vi "IO Initial.vi"(8 "error in (no error)":errorcluster, 10 "CardType":u16[](array[ring])=[16, 37] items=["PCI-7230"=6, "PCI-7432"=16, "PCI-7433"=17, "PCI-7434"=18, "PCI-7442"=37]) -> (0 "error out":errorcluster, 2 "IO f":i16[](array[numeric]))   [LabVIEW 2017]
uses:
  <vilib>/Utility/file.llb/Read From Spreadsheet File (string).vi
  Adlink IO/Adlink IO.lvlib
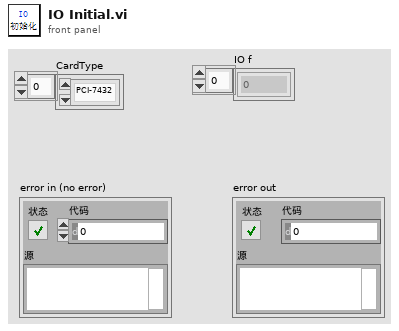
[diagram p1: front panel]
types:
  T1 = cluster{"DI dev":i32[], "DI line":i32[], "Port":i32[], "DO dev":i32[], "DO line":i32[], "IO Data":string[][], "IO f":i16[]}
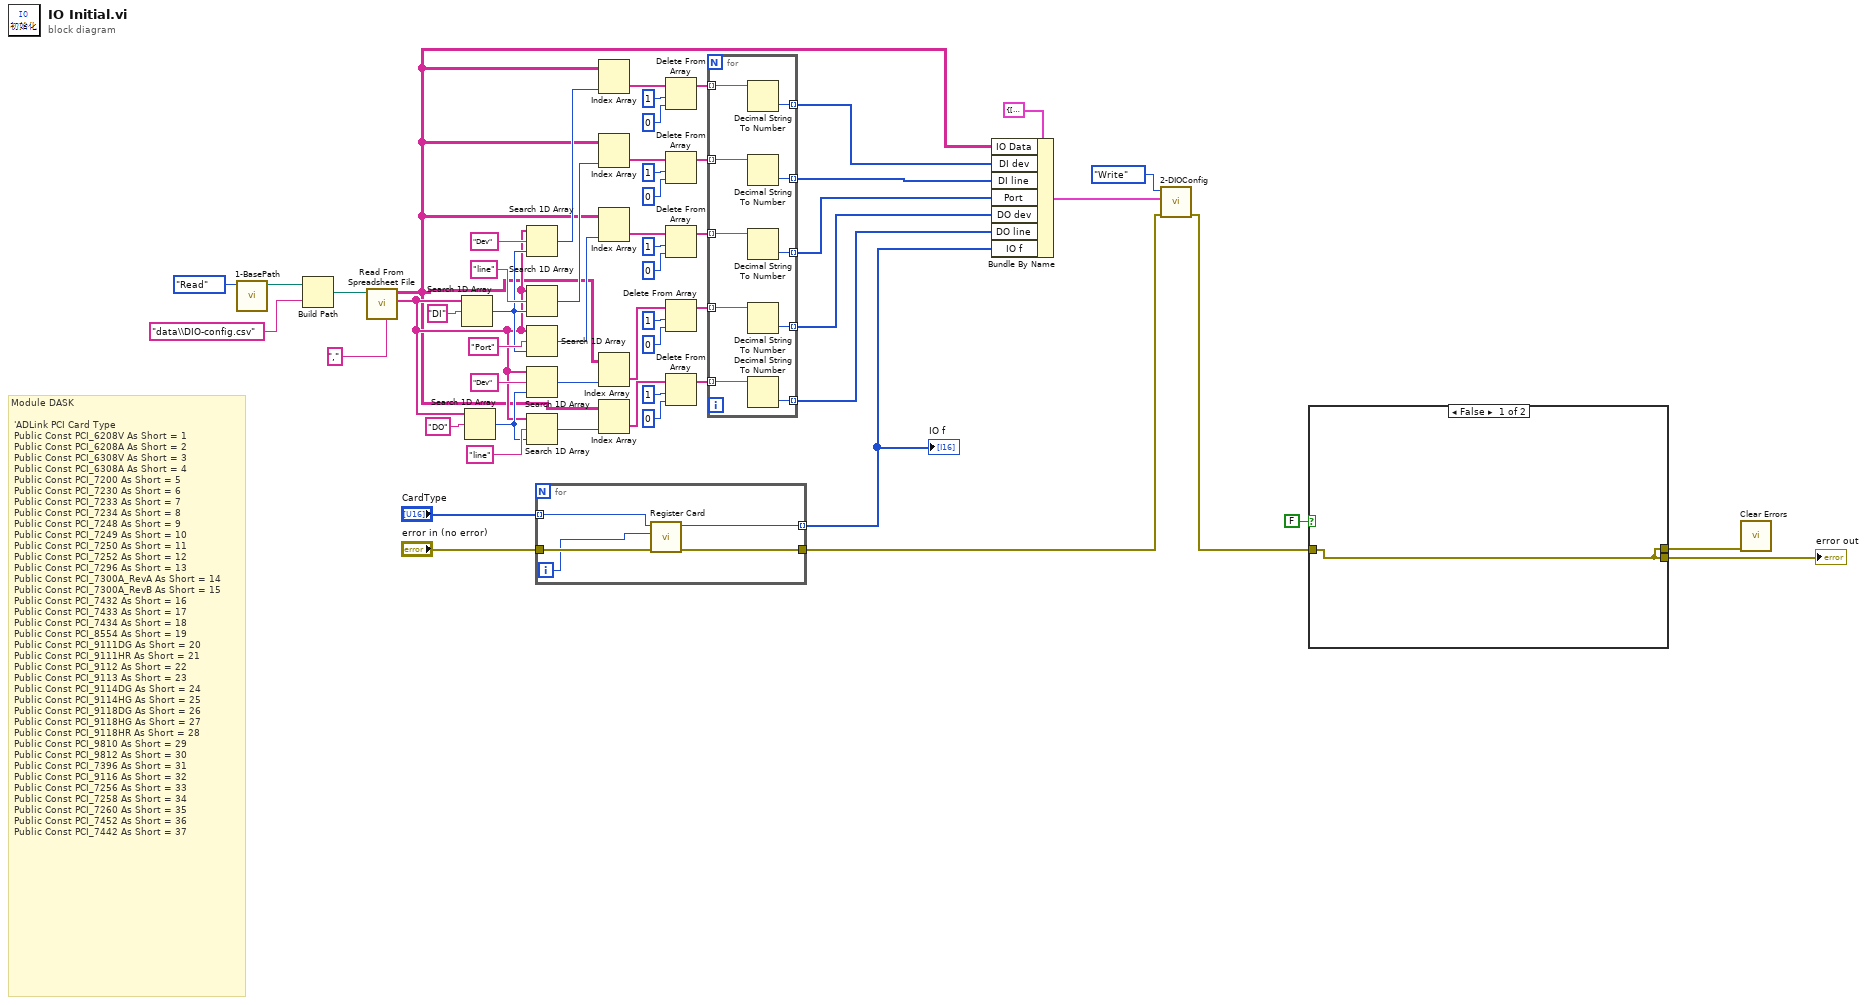
[diagram p0: block diagram]
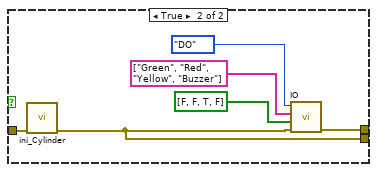
[diagram p2: hidden frame]
diagram:
  # "Module DASK\n\t\n\t'ADLink PCI Card Type\n\tPublic Const PCI_6208V As Short = 1\n\tPublic Const PCI_6208A As Short = 2\n\tPublic Const PCI_6308V As Short = 3\n\tPublic Const PCI_6308A As Short = 4\n\tPublic Const PCI_7200 As Short = 5\n\tPublic Const PCI_7230 As Short = 6\n\tPublic Const PCI_7233 As Short = 7\n\tPublic Const PCI_7234 As Short = 8\n\tPublic Const PCI_7248 As Short = 9\n\tPublic Const PCI_7249 As Short = 10\n\tPublic Const PCI_7250 As Short = 11\n\tPublic Const PCI_7252 As Short = 12\n\tPublic Const PCI_7296 As Short = 13\n\tPublic Const PCI_7300A_RevA As Short = 14\n\tPublic Const PCI_7300A_RevB As Short = 15\n\tPublic Const PCI_7432 As Short = 16\n\tPublic Const PCI_7433 As Short = 17\n\tPublic Const PCI_7434 As Short = 18\n\tPublic Const PCI_8554 As Short = 19\n\tPublic Const PCI_9111DG As Short = 20\n\tPublic Const PCI_9111HR As Short = 21\n\tPublic Const PCI_9112 As Short = 22\n\tPublic Const PCI_9113 As Short = 23\n\tPublic Const PCI_9114DG As Short = 24\n\tPublic Const PCI_9114HG As Short = 25\n\tPublic Const PCI_9118DG As Short = 26\n\tPublic Const PCI_9118HG As Short = 27\n\tPublic Const PCI_9118HR As Short = 28\n\tPublic Const PCI_9810 As Short = 29\n\tPublic Const PCI_9812 As Short = 30\n\tPublic Const PCI_7396 As Short = 31\n\tPublic Const PCI_9116 As Short = 32\n\tPublic Const PCI_7256 As Short = 33\n\tPublic Const PCI_7258 As Short = 34\n\tPublic Const PCI_7260 As Short = 35\n\tPublic Const PCI_7452 As Short = 36\n\tPublic Const PCI_7442 As Short = 37"
  n1 = call "1-BasePath.vi"("Step"=enum16{"Initial", "Write", "Read"}."Read") -> ("Path Out"=w8:path)  [unwired: 9 in, 1 out]
  n2 = Build Path(base path=w8, name or relative path="data\\DIO-config.csv" ("名称或相对路径")) -> (appended path=w7:path)
  n3 = call-poly <vilib>:"Read From Spreadsheet File.vi"("delimiter (\\t)"="," ("delimiter (\\t)"), "file path (dialog if empty)"=w7) -> ("first row"=w21:string[], "all rows"=w13:string[][])  [unwired: 5 in, 3 out]
  n4 = Search 1D Array(1D array=w21, element="DI" ("元素")) -> (index of element=w22:i32)  [unwired: 1 in]
  n5 = Search 1D Array(1D array=w21, element="DO" ("元素")) -> (index of element=w24:i32)  [unwired: 1 in]
  n6 = Search 1D Array(1D array=w21, element="Dev" ("元素"), start index (0)=w22) -> (index of element=w27:i32)
  n7 = Search 1D Array(1D array=w21, element="line" ("元素"), start index (0)=w22) -> (index of element=w34:i32)
  n8 = Search 1D Array(1D array=w21, element="Port" ("元素"), start index (0)=w22) -> (index of element=w40:i32)
  n9 = Search 1D Array(1D array=w21, element="Dev" ("元素"), start index (0)=w24) -> (index of element=w42:i32)
  n10 = Search 1D Array(1D array=w21, element="line" ("元素"), start index (0)=w24) -> (index of element=w51:i32)
  n11 = for {
    tunnel: [w59] -> w55 mode=indexing
    tunnel: [w62] -> w6
    tunnel: "error in (no error)" -> [w61]
    tunnel: "CardType" -> [w60] mode=indexing
    i -> [w58]
    n12 = call "Register Card.vi"("error in (no error)"=w61, "card_num"=w58, "CardType"=w60) -> ("error out"=w62:errorcluster, "function return"=w59:i16)  [unwired: 7 in]
  }
  "IO f" <- w55
  n13 = Index Array(array=w13, index (col)=w27) -> (element=w28:string[])  [unwired: 1 in]
  n14 = Index Array(array=w13, index (col)=w34) -> (element=w33:string[])  [unwired: 1 in]
  n15 = Index Array(array=w13, index (col)=w40) -> (element=w37:string[])  [unwired: 1 in]
  n16 = Index Array(array=w13, index (col)=w42) -> (element=w44:string[])  [unwired: 1 in]
  n17 = Index Array(array=w13, index (col)=w51) -> (element=w50:string[])  [unwired: 1 in]
  n18 = Delete From Array(array=w28, length=1 ("长度"), index=0 ("索引")) -> (array with subset deleted=w20:string[])  [unwired: 1 out]
  n19 = Delete From Array(array=w33, length=1 ("长度"), index=0 ("索引")) -> (array with subset deleted=w19:string[])  [unwired: 1 out]
  n20 = Delete From Array(array=w37, length=1 ("长度"), index=0 ("索引")) -> (array with subset deleted=w18:string[])  [unwired: 1 out]
  n21 = Delete From Array(array=w44, length=1 ("索引"), index=0 ("索引")) -> (array with subset deleted=w47:string[])  [unwired: 1 out]
  n22 = Delete From Array(array=w50, length=1 ("索引"), index=0 ("索引")) -> (array with subset deleted=w53:string[])  [unwired: 1 out]
  n23 = for {
    tunnel: w47 -> [w72] mode=indexing
    tunnel: w53 -> [w70] mode=indexing
    tunnel: [w71] -> w14 mode=indexing
    tunnel: [w69] -> w5 mode=indexing
    tunnel: w20 -> [w68] mode=indexing
    tunnel: w19 -> [w67] mode=indexing
    tunnel: w18 -> [w66] mode=indexing
    tunnel: [w65] -> w17 mode=indexing
    tunnel: [w64] -> w16 mode=indexing
    tunnel: [w63] -> w15 mode=indexing
    n24 = Decimal String To Number(string=w68) -> (number=w65:i32)  [unwired: 2 in, 1 out]
    n25 = Decimal String To Number(string=w67) -> (number=w64:i32)  [unwired: 2 in, 1 out]
    n26 = Decimal String To Number(string=w66) -> (number=w63:i32)  [unwired: 2 in, 1 out]
    n27 = Decimal String To Number(string=w72) -> (number=w71:i32)  [unwired: 2 in, 1 out]
    n28 = Decimal String To Number(string=w70) -> (number=w69:i32)  [unwired: 2 in, 1 out]
  }
  n29 = Bundle By Name(cluster=T1 {"DI dev"=[], "DI line"=[], "Port"=[], "DO dev"=[], "DO line"=[], "IO Data"=[], "IO f"=[]} ("IO pra in"), "IO Data"=w13, "DI dev"=w17, "DI line"=w16, "Port"=w15, "DO dev"=w14, "DO line"=w5, "IO f"=w55) -> (w12:T1)
  n30 = call "2-DIOConfig.vi"("error in (no error)"=w6, "DIO pra in"=w12, "Step"=enum16{"Initial", "Write", "Read"}."Write") -> ("error out"=w4:errorcluster)  [unwired: 7 in, 1 out]
  n31 = case shown="False" FALSE {
    tunnel: w4 -> [w73 w79]
    tunnel: [w73 w75] -> w3
    tunnel: [w73 w74] -> w2
    frame False {
    }
    frame True {
      n32 = call "ini_Cylinder.vi"("error IO"=w79) -> ("error out"=w74:errorcluster)  [unwired: 10 in]
      n33 = call "IO.vi"("错误常量"=w74, "DO DATA"=bool[] [FALSE, FALSE, TRUE, FALSE], "IO Name"=string[] ["Green", "Red", "Yellow", "Buzzer"], "IO?"=enum16{"DI", "DO"}."DO") -> ("error out"=w75:errorcluster)  [unwired: 5 in, 2 out]
    }
  }
  "error out" <- w2
  n34 = call <vilib>:"Clear Errors.vi"("error in (no error)"=w3) -> ()  [unwired: 5 in, 2 out]
